vi "Search and ReplaceTest Info Array.vi"(9 "Search Parameter  Table":string[][](array[string]), 11 "Parameter Table":string[][](array[string])) -> (3 "New Parameter Table":string[][](array[string]))   [LabVIEW 2010]
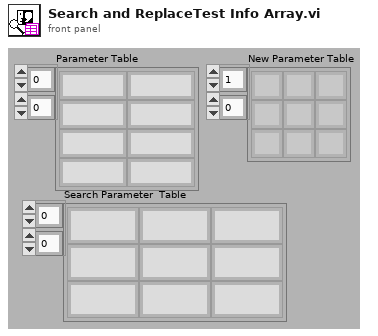
[diagram p1: front panel]
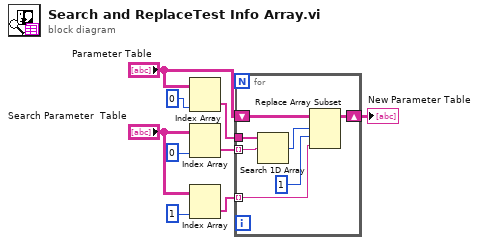
[diagram p0: block diagram]
diagram:
  n1 = Index Array(array="Parameter Table", index (col)=0 ("index (row)")) -> (element=w2:string[])  [unwired: 1 in]
  n2 = Index Array(array="Search Parameter  Table", index (col)=0 ("disabled index (col)")) -> (element=w7:string[])  [unwired: 1 in]
  n3 = Index Array(array="Search Parameter  Table", index (col)=1 ("disabled index (col)")) -> (element=w4:string[])  [unwired: 1 in]
  n4 = for {
    shift-right: [w13] -> w9
    shift-left: "Parameter Table" -> [w16]
    tunnel: w7 -> [w10] mode=indexing
    tunnel: w4 -> [w12] mode=indexing
    tunnel: w2 -> [w11]
    n5 = Search 1D Array(1D array=w11, element=w10) -> (index of element=w15:i32)  [unwired: 1 in]
    n6 = Replace Array Subset(array=w16, new element=w12, index (row)=w15, index (col)=1 ("disabled index (col)")) -> (w13:string[][])
  }
  "New Parameter Table" <- w9
